vi "Alarm Condition.vi"(0 "VISA resource name":refnum<visa-resource-name>, 5 "Channel (1)":i32=1 min=1 max=16 step=1, 11 "error in (no error)":errorcluster) -> (4 "VISA resource name out":refnum<visa-resource-name>, 8 "Alarm High Status":bool, 10 "Alarm Low Status":bool, 15 "error out":errorcluster)   [LabVIEW 2025, in "Lake Shore Cryotronics 370.lvlib"]
doc: "This VI indicates the status of the alarm for the selected channel."
uses:
  Lake Shore Cryotronics 370.lvlib
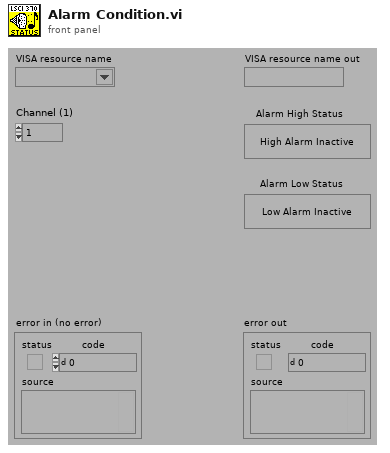
[diagram p1: front panel]
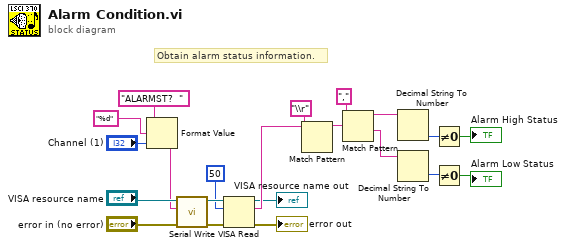
[diagram p0: block diagram]
diagram:
  # "Obtain alarm status information."
  n1 = Format Value(string ("")="ALARMST?  ", format string="%d", value (0)="Channel (1)") -> (output string=w3:string)
  n2 = call "Serial Write.vi"("error in (no error)"="error in (no error)", "Write Buffer (\"\")"=w3, "VISA resource name"="VISA resource name") -> ("error out"=w20:errorcluster, "VISA resource name out"=w21:refnum<visa-resource-name>)  [unwired: 6 in, 1 out]
  n3 = VISA Read(VISA resource name=w21, byte count=50, error in (no error)=w20) -> (VISA resource name out=→"VISA resource name out":refnum<visa-resource-name>, read buffer=w18:string, error out=→"error out":errorcluster)  [unwired: 1 out]
  n4 = Match Pattern(string=w18, regular expression="\\r") -> (before substring=w15:string)  [unwired: 1 in, 3 out]
  n5 = Match Pattern(string=w15, regular expression=",") -> (before substring=w14:string, after substring=w13:string)  [unwired: 1 in, 2 out]
  n6 = Decimal String To Number(string=w14) -> (number=w12:i32)  [unwired: 2 in, 1 out]
  n7 = Decimal String To Number(string=w13) -> (number=w11:i32)  [unwired: 2 in, 1 out]
  n8 = Not Equal To 0?(x=w12) -> (x != 0?=→"Alarm High Status":bool)
  n9 = Not Equal To 0?(x=w11) -> (x != 0?=→"Alarm Low Status":bool)
